vi "NI.History (Path).vi"(1 "value in":path) -> (0 "Stop?":bool)   [LabVIEW 2020]
doc: "Displays the value of the 32-bit signed integer numeric control and allows conditional breakpoints."
uses:
  <vilib>/Utility/miscctls.llb/LVRowAndColumnUnsignedTypeDef.ctl
panel:
  out "History":i32(listbox)=-1
  in  "reset":bool
  # "* Changes take effect the next time the probe runs."
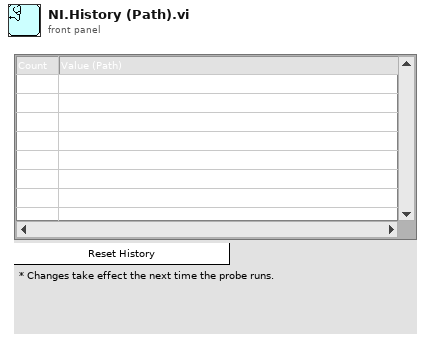
[diagram p1: front panel]
types:
  T1 = typedef "LVRowAndColumnUnsignedTypeDef.ctl" = cluster{"Row":u32, "Column":u32}
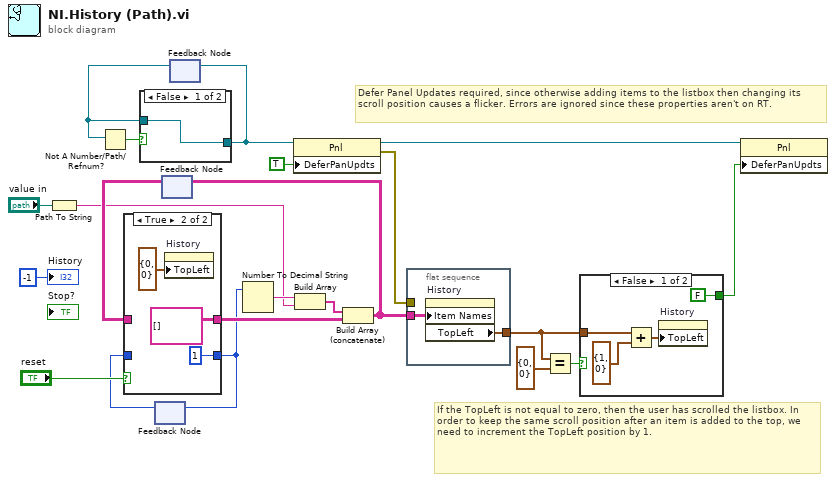
[diagram p0: block diagram]
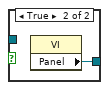
[diagram p3: hidden frame]
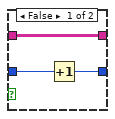
[diagram p4: hidden frame]
diagram:
  # "If the TopLeft is not equal to zero, then the user has scrolled the listbox. In order to keep the same scroll position after an item is added to the top, we need to increment the TopLeft position by 1."
  # "Defer Panel Updates required, since otherwise adding items to the listbox then changing its scroll position causes a flicker. Errors are ignored since these properties aren't on RT."
  n1 = Path To String(path="value in") -> (string=w11:string)
  n2 = feedback #1() -> (w15:i32)  [unwired: 1 in]
  n3 = feedback #2() -> (w14:string[][])  [unwired: 1 in]
  n4 = case shown="True" "reset" {
    tunnel: w14 -> [w24 _]
    tunnel: w15 -> [w23 _]
    tunnel: [w24 string[][] []] -> w19
    tunnel: [w22 1] -> w16
    frame False {
      n5 = Increment(x=w23) -> (x+1=w22:i32)
    }
    frame True {
      n6 = property on="History" class="MCListbox (strict)"("TopLeft"=T1 {"Row"=0, "Column"=0} ("Top Left Visible Cell")) -> ()  [unwired: 2 in, 2 out]
    }
  }
  n7 = feedback-in #1(w16) -> ()
  n8 = feedback #3() -> (w7:refnum<vi>)  [unwired: 1 in]
  n9 = Not A Number/Path/Refnum?(number/path/refnum=w7) -> (NaN/Path/Refnum?=w8:bool)
  n10 = case shown="False" w8 {
    tunnel: [w28 w29] -> w9
    tunnel: w7 -> [w28 _]
    frame False {
    }
    frame True {
      n11 = property class="VI"() -> ("Panel"=w29:refnum<vi>)  [unwired: 2 in, 2 out]
    }
  }
  n12 = feedback-in #3(w9) -> ()
  n13 = Number To Decimal String(number=w16) -> (decimal integer string=w17:string)  [unwired: 1 in]
  n14 = property class="Pnl"(reference=w9, "DeferPanUpdts"=TRUE ("Defer Panel Updates")) -> (reference out=w6:refnum<vi>, error out=w5:errorcluster)  [unwired: 1 in]
  n15 = Build Array(w17, w11) -> (w18:string[])
  n16 = Build Array (concatenate)(w18, w19) -> (w13:string[][])
  n17 = feedback-in #2(w13) -> ()
  n18 = flat-sequence {
    tunnel: w13 -> [w31]
    tunnel: w5 -> [_]
    tunnel: [w30] -> w2
    frame #0 {
      n19 = property on="History" class="MCListbox (strict)"("Item Names"=w31) -> ("TopLeft"=w30:T1)  [unwired: 2 in, 2 out]
    }
  }
  n20 = Equal?(x=w2, y=T1 {"Row"=0, "Column"=0} ("Top Left Visible Cell")) -> (x = y?=w3:bool)
  n21 = case shown="False" w3 {
    tunnel: w2 -> [w35 _]
    tunnel: [FALSE ("Defer Panel Updates") _] -> w1
    frame False {
      n22 = Add(x=w35, y=T1 {"Row"=1, "Column"=0}) -> (x+y=w33:T1)
      n23 = property on="History" class="MCListbox (strict)"("TopLeft"=w33) -> ()  [unwired: 2 in, 2 out]
    }
    frame True {
    }
  }
  n24 = property class="Pnl"(reference=w6, "DeferPanUpdts"=w1) -> ()  [unwired: 1 in, 2 out]
  "History" <- -1 ("History of Values")
